vi "Set Multi Track Scan.vi"(0 "trackHeight":i32, 1 "trackHBinning":i32, 2 "trackGap":i32, 3 "trackSkip":i32, 5 "numberTracks":i32, 7 "iSIHStart":i32, 9 "iSIHEnd":i32, 12 "trackVBinning":i32, 13 "trackOffset":i32, 14 "numberSubFrames":i32) -> (4 "function return":u32)   [LabVIEW 2018, in "Copy of Andor SDK.lvlib"]
doc: "EXPNETTYPE unsigned int WINAPI SetMultiTrackScan(int trackHeight, int numberTracks, int iSIHStart, int iSIHEnd, int trackHBinning, int trackVBinning, int trackGap, int trackOffset, int trackSkip, int numberSubFrames);"
uses:
  Copy of Andor SDK.lvlib
  <userlib>/Andor SDK/ATMCD32D.dll
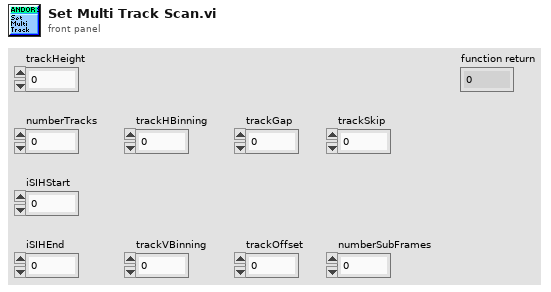
[diagram p1: front panel]
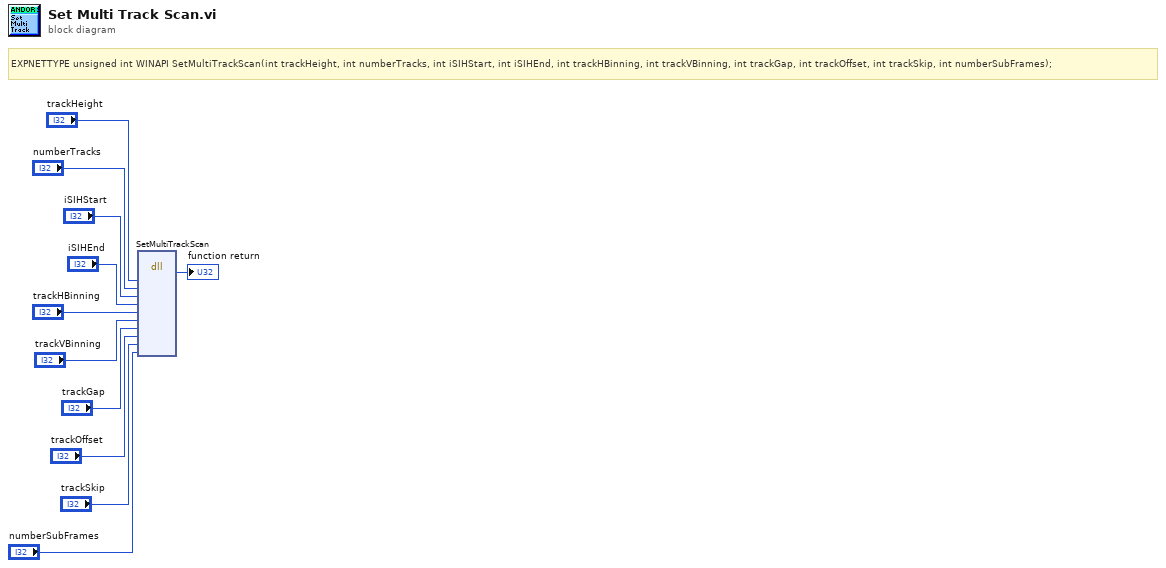
[diagram p0: block diagram]
diagram:
  # "EXPNETTYPE unsigned int WINAPI SetMultiTrackScan(int trackHeight, int numberTracks, int iSIHStart, int iSIHEnd, int trackHBinning, int trackVBinning, int trackGap, int trackOffset, int trackSkip, int numberSubFrames);"
  n1 = dll-call lib="C:/Program Files (x86)/National Instruments/LabVIEW 2018/user.lib/Andor SDK/ATMCD32D.*" fn="SetMultiTrackScan"("trackHeight"="trackHeight", "numberTracks"="numberTracks", "iSIHStart"="iSIHStart", "iSIHEnd"="iSIHEnd", "trackHBinning"="trackHBinning", "trackVBinning"="trackVBinning", "trackGap"="trackGap", "trackOffset"="trackOffset", "trackSkip"="trackSkip", "numberSubFrames"="numberSubFrames") -> (→"function return":u32)  [unwired: 13 in, 2 out]
